vi "INI.GetSettings.vi"(8 "error in (no error)":errorcluster, 10 "INI Folder Location":path, 11 "State Variables":T1={"Events.State"=refnum, "Events.Test Result"=refnum, "Events.Progress"=refnum, "INI.Settings"={"Build Location"=path "C:/Simple Sequence Editor/SequenceRepo", "LoggingLocation"=path "", "Sequence.AbortChannel"="", "Sequence.IterationInfoChannel"="", "Sequence.DurationChannel"="", "Sequence.StepInfoChannel"="", "Sequence.SkipChannel"="", "PlotChannels"=[], "Sequence.InitializeScript"=path "C:/Simple Sequence Editor/SequenceRepo", "Sequence.CleanupScript"=path "", "Log.DefaultRate"=0.0}, "NIVS.AlarmManager"=refnum, "NIVS.BaseLogPath"=path "", "NIVS.DataLogManagerRef"=refnum, "NIVS.DataLogSpecRef"=refnum, "NIVS.Deployed"=FALSE, "NIVS.Events"={"SequenceEvent"=refnum, "SystemChangeEvent"=refnum, "WorkspaceEvent"=refnum}, "NIVS.GatewayIPAddress"="", "NIVS.DataLogGUID"="", "NIVS.ProfileCallback"=refnum, "NIVS.ProfileRef"=refnum, "NIVS.SequenceState"=enum."Idle", "NIVS.SystemDefinitionFile"=path "", "NIVS.SystemStateRefs"={"CustDatRef"=refnum, "EvtRef"=refnum, "Target State User Event"=refnum}, "NIVS.WorkspaceManager"=refnum, "NIVS.EventLogGUID"="", "NIVS.EventLogManagerRef"=refnum, "NIVS.EventLogSpecRef"=refnum, "NIVS.BaseToolPath"=path "", "Restart.Path"=path "", "Sequence.#ofColumns"=0, "Sequence.Iterations"=0, "Sequence.Channels"=[], "Sequence.ValidConfig?"=FALSE, "Station.ID"="", "UDP.Queue"=refnum, "UI.Abort"=refnum, "UI.Alarms"=refnum, "UI.Apply"=refnum, "UI.Back"=refnum, "UI.BaseFileName"=refnum, "UI.CurrentIteration"=refnum, "UI.CurrentStep"=refnum, "UI.CyclicFrequency"=refnum, "UI.Description"=refnum, "UI.DelayTime"=refnum, "UI.DisableAlarms"=refnum, "UI.Duration"=refnum, "UI.EnableLogging"=refnum, "UI.EnableState"=refnum, "UI.High"=refnum, "UI.LogChannels"=refnum, "UI.Low"=refnum, "UI.MonitoredVariable"=refnum, "UI.Next"=refnum, "UI.NumberOfCycles"=refnum, "UI.OperatorName"=refnum, "UI.Pause"=refnum, "UI.Profile"=refnum, "UI.Revert"=refnum, "UI.Skip"=refnum, "UI.Start"=refnum, "UI.StartIteration"=refnum, "UI.StartStep"=refnum, "UI.TabControl"=refnum, "UI.TotalIterations"=refnum, "UI.WaveformDefinition"=refnum, "UI.WaveformPreview"=refnum, "UI.WorkOrderNumber"=refnum, "UI.Chart"=refnum, "UI.Status"=refnum, "UI.DataView"=refnum, "UI.Table"=refnum, "UI.Multihead"=refnum, "UI.ToolTab"=refnum, "UI.Result"=refnum, "UI.Log Path"=refnum, "UI.ReportPath"=refnum, "UI.RestartPath"=refnum, "UI.AlarmLog"=refnum}) -> (0 "error out":errorcluster, 3 "INI.Settings":T2={"Build Location"=path "C:/Simple Sequence Editor/SequenceRepo", "LoggingLocation"=path "", "Sequence.AbortChannel"="", "Sequence.IterationInfoChannel"="", "Sequence.DurationChannel"="", "Sequence.StepInfoChannel"="", "Sequence.SkipChannel"="", "PlotChannels"=[], "Sequence.InitializeScript"=path "C:/Simple Sequence Editor/SequenceRepo", "Sequence.CleanupScript"=path "", "Log.DefaultRate"=0.0})   [LabVIEW 2015, in "Single Station Execution.lvlib"]
uses:
  Single Station Execution.lvlib
  Types/INI.Settings.ctl
  Types/Main.StateVariables.ctl
  <vilib>/NI Veristand/Execution/AlarmManager/AlarmManagerAPI.ctl
  NationalInstruments.VeriStand.ClientAPI
  <vilib>/NI Veristand/Execution/DataLogging/IDataLogging Ref.ctl
  <vilib>/NI Veristand/Execution/DataLogging/DataLoggingSpecification Ref.ctl
  Types/Execute.UserEventRefs.ctl
  <vilib>/NI Veristand/Execution/Workspace/SystemStateRegEventRef.ctl
  <vilib>/NI Veristand/Execution/Workspace/Target State Info.ctl
  <vilib>/NI Veristand/Execution/Workspace/Target State.ctl
  Types/Execution.SequenceState.ctl
  <vilib>/NI Veristand/Execution/Workspace/SystemStateEventRef.ctl
  <vilib>/NI Veristand/Execution/Workspace/WorkspaceAPI.ctl
  Types/UDPEngine.QueueCluster.ctl
  Types/UDPEngine.State.ctl
  Main.Constants.vi
  <vilib>/Utility/config.llb/Read Key (Path).vi
  <vilib>/Utility/config.llb/Write Key (Path).vi
  <vilib>/Utility/config.llb/Read Key (Double).vi
  <vilib>/Utility/config.llb/Write Key (Double).vi
  <vilib>/Utility/config.llb/Read Key (String).vi
  <vilib>/Utility/config.llb/Write Key (String).vi
  <vilib>/Utility/config.llb/NI_LVConfig.lvlib
  <vilib>/NI Veristand/Execution/Workspace/NI_VS Workspace ExecutionAPI.lvlib
  <vilib>/NI Veristand/Execution/DataLogging/NI_VS Data Logging API.lvlib
  <vilib>/NI Veristand/Execution/AlarmManager/NI_VS AlarmManager ExecutionAPI.lvlib
  NationalInstruments.VeriStand.RealTimeSequenceDefinitionApi
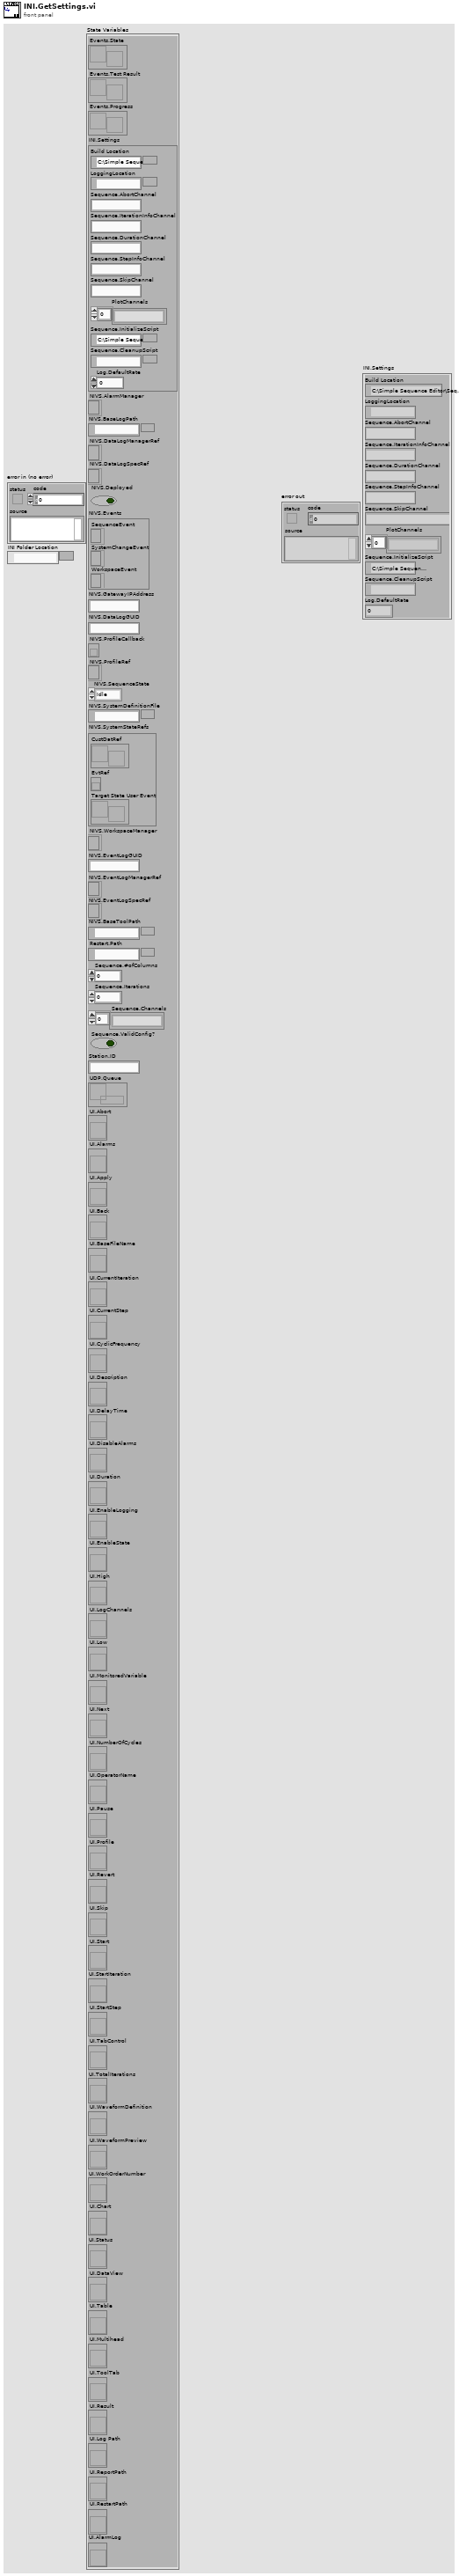
[diagram p1: front panel]
types:
  T1 = typedef "Single Station Execution.lvlib/Main.StateVariables.ctl" = cluster{"Events.State":refnum<user-event>, "Events.Test Result":refnum<user-event>, "Events.Progress":refnum<user-event>, "INI.Settings":T2, "NIVS.AlarmManager":T3, "NIVS.BaseLogPath":path, "NIVS.DataLogManagerRef":T4, "NIVS.DataLogSpecRef":T5, "NIVS.Deployed":bool, "NIVS.Events":T6, "NIVS.GatewayIPAddress":string, "NIVS.DataLogGUID":string, "NIVS.ProfileCallback":refnum<k27>, "NIVS.ProfileRef":refnum<k24>, "NIVS.SequenceState":T8, "NIVS.SystemDefinitionFile":path, "NIVS.SystemStateRefs":T9, "NIVS.WorkspaceManager":T10, "NIVS.EventLogGUID":string, "NIVS.EventLogManagerRef":T4, "NIVS.EventLogSpecRef":T5, "NIVS.BaseToolPath":path, "Restart.Path":path, "Sequence.#ofColumns":i32, "Sequence.Iterations":u32, "Sequence.Channels":string[], "Sequence.ValidConfig?":bool, "Station.ID":string, "UDP.Queue":refnum<queue>, "UI.Abort":refnum<vi>, "UI.Alarms":refnum<vi>, "UI.Apply":refnum<vi>, "UI.Back":refnum<vi>, "UI.BaseFileName":refnum<vi>, "UI.CurrentIteration":refnum<vi>, "UI.CurrentStep":refnum<vi>, "UI.CyclicFrequency":refnum<vi>, "UI.Description":refnum<vi>, "UI.DelayTime":refnum<vi>, "UI.DisableAlarms":refnum<vi>, "UI.Duration":refnum<vi>, "UI.EnableLogging":refnum<vi>, "UI.EnableState":refnum<vi>, "UI.High":refnum<vi>, "UI.LogChannels":refnum<vi>, "UI.Low":refnum<vi>, "UI.MonitoredVariable":refnum<vi>, "UI.Next":refnum<vi>, "UI.NumberOfCycles":refnum<vi>, "UI.OperatorName":refnum<vi>, "UI.Pause":refnum<vi>, "UI.Profile":refnum<vi>, "UI.Revert":refnum<vi>, "UI.Skip":refnum<vi>, "UI.Start":refnum<vi>, "UI.StartIteration":refnum<vi>, "UI.StartStep":refnum<vi>, "UI.TabControl":refnum<vi>, "UI.TotalIterations":refnum<vi>, "UI.WaveformDefinition":refnum<vi>, "UI.WaveformPreview":refnum<vi>, "UI.WorkOrderNumber":refnum<vi>, "UI.Chart":refnum<vi>, "UI.Status":refnum<vi>, "UI.DataView":refnum<vi>, "UI.Table":refnum<vi>, "UI.Multihead":refnum<vi>, "UI.ToolTab":refnum<vi>, "UI.Result":refnum<vi>, "UI.Log Path":refnum<vi>, "UI.ReportPath":refnum<vi>, "UI.RestartPath":refnum<vi>, "UI.AlarmLog":refnum<vi>}
  T2 = typedef "Single Station Execution.lvlib/INI.Settings.ctl" = cluster{"Build Location":path, "LoggingLocation":path, "Sequence.AbortChannel":string, "Sequence.IterationInfoChannel":string, "Sequence.DurationChannel":string, "Sequence.StepInfoChannel":string, "Sequence.SkipChannel":string, "PlotChannels":string[], "Sequence.InitializeScript":path, "Sequence.CleanupScript":path, "Log.DefaultRate":dbl}
  T3 = typedef "NI_VS AlarmManager ExecutionAPI.lvlib/AlarmManagerAPI.ctl" = refnum<k24>
  T4 = typedef "NI_VS Data Logging API.lvlib/IDataLogging Ref.ctl" = refnum<k24>
  T5 = typedef "NI_VS Data Logging API.lvlib/DataLoggingSpecification Ref.ctl" = refnum<k24>
  T6 = typedef "Single Station Execution.lvlib/Execute.UserEventRefs.ctl" = cluster{"SequenceEvent":refnum<event-registration>, "SystemChangeEvent":T7, "WorkspaceEvent":refnum<event-registration>}
  T7 = typedef "NI_VS Workspace ExecutionAPI.lvlib/SystemStateRegEventRef.ctl" = refnum<event-registration>
  T8 = typedef "Single Station Execution.lvlib/Execution.SequenceState.ctl" = enum16{"Idle", "Initializing", "Running", "Paused", "Finalizing", "Complete"}
  T9 = typedef "NI_VS Workspace ExecutionAPI.lvlib/SystemStateEventRef.ctl" = cluster{"CustDatRef":refnum<user-event>, "EvtRef":refnum<k27>, "Target State User Event":refnum<user-event>}
  T10 = typedef "NI_VS Workspace ExecutionAPI.lvlib/WorkspaceAPI.ctl" = refnum<k24>
  T11 = typedef "NI_LVConfig.lvlib/Config Data RefNum.ctl" = refnum<k1>
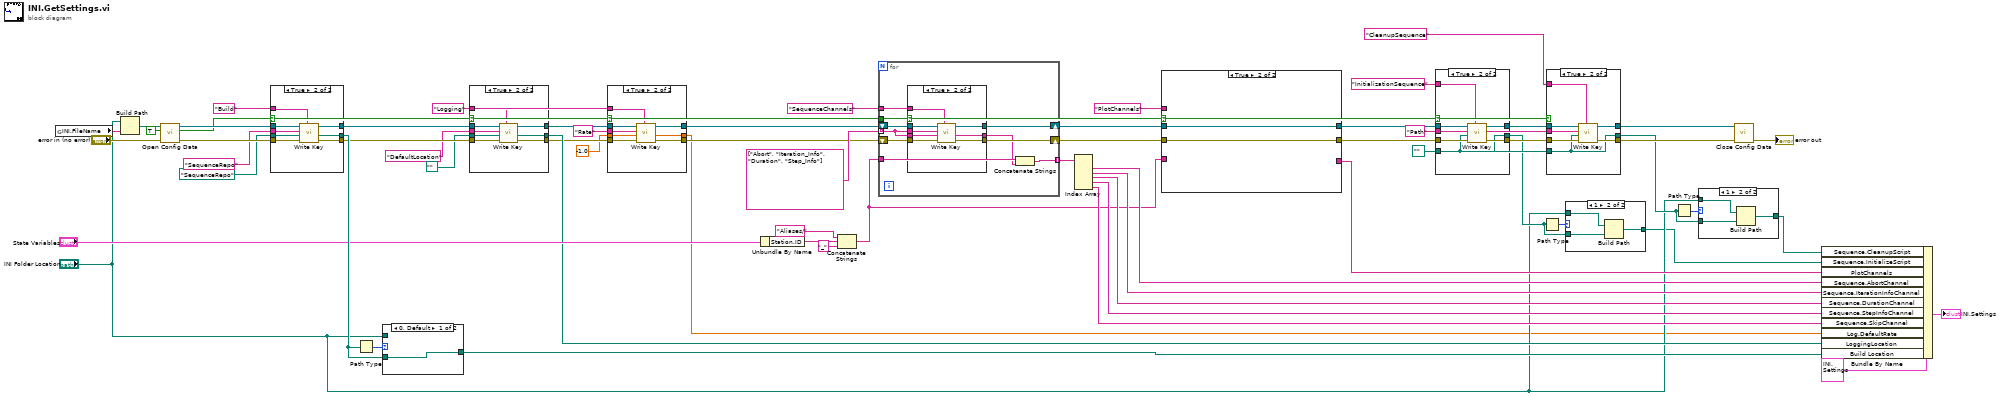
[diagram p0: block diagram]
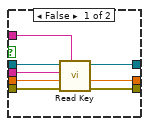
[diagram p2: hidden frame]
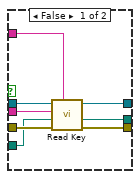
[diagram p5: hidden frame]
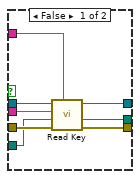
[diagram p6: hidden frame]
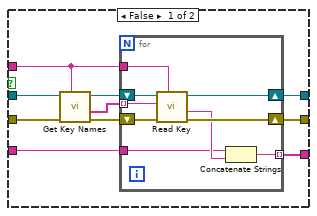
[diagram p7: hidden frame]
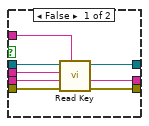
[diagram p8: hidden frame]
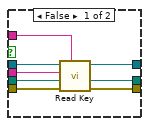
[diagram p9: hidden frame]
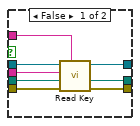
[diagram p10: hidden frame]
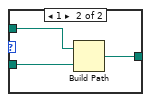
[diagram p11: hidden frame]
diagram:
  w22 = path "" ("default value")
  w18 = "Path" ("section")
  w6 = "Logging" ("section")
  n1 = global read "Main.Constants.vi" "INI.FileName"() -> (w55:string)
  n2 = Build Path(base path="INI Folder Location", name or relative path=w55) -> (appended path=w56:path)
  n3 = call <vilib>:"Open Config Data.vi"("error in (no error)"="error in (no error)", "create file if necessary (T)"=TRUE, "configuration file path"=w56) -> ("error out"=w62:errorcluster, "file created?"=w7:bool, "refnum"=w63:T11)  [unwired: 6 in]
  n4 = case shown="True" w7 {
    tunnel: w63 -> [w71 w76]
    tunnel: w62 -> [w70 w78]
    tunnel: [w69 w74] -> w48
    tunnel: [w68 w72] -> w46
    tunnel: "Build" ("section") -> [w67 w75]
    tunnel: "SequenceRepo" ("key") -> [w66 w77]
    tunnel: path "SequenceRepo" ("default value") -> [w65 w73]
    tunnel: [w64 w73] -> w57
    frame False {
      n5 = call-poly <vilib>:"Read Key.vi"("section"=w67, "error in (no error)"=w70, "default value"=w65, "key"=w66, "refnum"=w71) -> ("error out"=w69:errorcluster, "value"=w64:path, "refnum out"=w68:T11)  [unwired: 3 in, 1 out]
    }
    frame True {
      n6 = call-poly <vilib>:"Write Key.vi"("section"=w75, "error in (no error)"=w78, "value"=w73, "key"=w77, "refnum"=w76) -> ("error out"=w74:errorcluster, "refnum out"=w72:T11)  [unwired: 4 in, 1 out]
    }
  }
  n7 = Path Type(1:w57) -> (0:w58:i16)
  n8 = case shown="0, Default" w58 {
    tunnel: w57 -> [w79 w82]
    tunnel: [w79 w81] -> w50
    tunnel: "INI Folder Location" -> [_ w80]
    frame 0, Default {
    }
    frame 1 {
      n9 = Build Path(base path=w80, name or relative path=w82) -> (appended path=w81:path)
    }
  }
  n10 = case shown="True" w7 {
    tunnel: w46 -> [w90 w95]
    tunnel: w48 -> [w89 w97]
    tunnel: [w88 w93] -> w9
    tunnel: [w87 w91] -> w3
    tunnel: w6 -> [w86 w94]
    tunnel: "DefaultLocation" ("key") -> [w85 w96]
    tunnel: path "" ("default value") -> [w84 w92]
    tunnel: [w83 w92] -> w32
    frame False {
      n11 = call-poly <vilib>:"Read Key.vi"("section"=w86, "error in (no error)"=w89, "default value"=w84, "key"=w85, "refnum"=w90) -> ("error out"=w88:errorcluster, "value"=w83:path, "refnum out"=w87:T11)  [unwired: 3 in, 1 out]
    }
    frame True {
      n12 = call-poly <vilib>:"Write Key.vi"("section"=w94, "error in (no error)"=w97, "value"=w92, "key"=w96, "refnum"=w95) -> ("error out"=w93:errorcluster, "refnum out"=w91:T11)  [unwired: 4 in, 1 out]
    }
  }
  n13 = case shown="True" w7 {
    tunnel: w3 -> [w105 w110]
    tunnel: w9 -> [w104 w112]
    tunnel: [w103 w108] -> w8
    tunnel: [w102 w106] -> w2
    tunnel: w6 -> [w101 w109]
    tunnel: "Rate" ("key") -> [w100 w111]
    tunnel: -1.0 -> [w99 w107]
    tunnel: [w98 w107] -> w1
    frame False {
      n14 = call-poly <vilib>:"Read Key.vi"("section"=w101, "error in (no error)"=w104, "default value"=w99, "key"=w100, "refnum"=w105) -> ("error out"=w103:errorcluster, "value"=w98:dbl, "refnum out"=w102:T11)  [unwired: 3 in, 1 out]
    }
    frame True {
      n15 = call-poly <vilib>:"Write Key.vi"("section"=w109, "error in (no error)"=w112, "value"=w107, "key"=w111, "refnum"=w110) -> ("error out"=w108:errorcluster, "refnum out"=w106:T11)  [unwired: 4 in, 1 out]
    }
  }
  n16 = Unbundle By Name("State Variables") -> ("Station.ID"=w33:string)
  n17 = Concatenate Strings("Aliases/" ("string"), w33, "_" ("string")) -> (w29:string)
  n18 = for {
    tunnel: w7 -> [w122]
    tunnel: "SequenceChannels" ("section") -> [w117]
    shift-right: [w120] -> w31
    shift-left: w8 -> [w121]
    shift-right: [w119] -> w28
    shift-left: w2 -> [w118]
    tunnel: string[] ["Abort", "Iteration_Info", "Duration", "Step_Info"] -> [w115] mode=indexing
    tunnel: [w113] -> w42 mode=indexing
    tunnel: w29 -> [w116]
    n19 = case shown="True" w122 {
      tunnel: w118 -> [w130 w135]
      tunnel: w121 -> [w129 w137]
      tunnel: [w128 w133] -> w120
      tunnel: [w127 w131] -> w119
      tunnel: w117 -> [w126 w134]
      tunnel: w115 -> [w125 w136]
      tunnel: w115 -> [w124 w132]
      tunnel: [w123 w132] -> w114
      frame False {
        n20 = call-poly <vilib>:"Read Key.vi"("section"=w126, "error in (no error)"=w129, "default value"=w124, "key"=w125, "refnum"=w130) -> ("error out"=w128:errorcluster, "value"=w123:string, "refnum out"=w127:T11)  [unwired: 3 in, 1 out]
      }
      frame True {
        n21 = call-poly <vilib>:"Write Key.vi"("section"=w134, "error in (no error)"=w137, "value"=w132, "key"=w136, "refnum"=w135) -> ("error out"=w133:errorcluster, "refnum out"=w131:T11)  [unwired: 4 in, 1 out]
      }
    }
    n22 = Concatenate Strings(w116, w114) -> (w113:string)
  }
  n23 = Index Array(array=w42) -> (element #1=w41:string, element #2=w37:string, element #3=w38:string, element #4=w39:string, element #5=w40:string)  [unwired: 5 in]
  n24 = case shown="True" w7 {
    tunnel: w28 -> [w146 w157]
    tunnel: w31 -> [w145 w156]
    tunnel: [w142 w156] -> w26
    tunnel: [w139 w157] -> w25
    tunnel: "PlotChannels" ("section") -> [w144 _]
    tunnel: w29 -> [w140 _]
    tunnel: [w138 _] -> w27
    frame False {
      n25 = call <vilib>:"Get Key Names.vi"("section"=w144, "error in (no error)"=w145, "refnum"=w146) -> ("error out"=w142:errorcluster, "key names"=w143:string[], "refnum out"=w141:T11)  [unwired: 5 in, 1 out]
      n26 = for {
        tunnel: w144 -> [w155]
        tunnel: w143 -> [w154] mode=indexing
        shift-right: [w151] -> w139
        shift-left: w141 -> [w152]
        shift-right: [w150] -> _
        shift-left: w142 -> [w153]
        tunnel: w140 -> [w148]
        tunnel: [w147] -> w138 mode=indexing
        n27 = call-poly <vilib>:"Read Key.vi"("section"=w155, "error in (no error)"=w153, "key"=w154, "refnum"=w152) -> ("error out"=w150:errorcluster, "value"=w149:string, "refnum out"=w151:T11)  [unwired: 4 in, 1 out]
        n28 = Concatenate Strings(w148, w149) -> (w147:string)
      }
    }
    frame True {
    }
  }
  n29 = case shown="True" w7 {
    tunnel: w26 -> [w165 w172]
    tunnel: [w164 w171] -> w23
    tunnel: w25 -> [w163 w169]
    tunnel: [w162 w170] -> w19
    tunnel: "InitializationSequence" ("section") -> [w161 w168]
    tunnel: w18 -> [w160 w167]
    tunnel: w22 -> [w159 w166]
    tunnel: [w158 w166] -> w12
    frame False {
      n30 = call-poly <vilib>:"Read Key.vi"("section"=w161, "error in (no error)"=w165, "default value"=w159, "key"=w160, "refnum"=w163) -> ("error out"=w164:errorcluster, "value"=w158:path, "refnum out"=w162:T11)  [unwired: 3 in, 1 out]
    }
    frame True {
      n31 = call-poly <vilib>:"Write Key.vi"("section"=w168, "error in (no error)"=w172, "value"=w166, "key"=w167, "refnum"=w169) -> ("error out"=w171:errorcluster, "refnum out"=w170:T11)  [unwired: 4 in, 1 out]
    }
  }
  n32 = Path Type(1:w12) -> (0:w13:i16)
  n33 = case shown="True" w7 {
    tunnel: w23 -> [w180 w187]
    tunnel: [w179 w186] -> w21
    tunnel: w19 -> [w178 w184]
    tunnel: [w177 w185] -> w20
    tunnel: "CleanupSequence" ("section") -> [w176 w183]
    tunnel: w18 -> [w175 w182]
    tunnel: w22 -> [w174 w181]
    tunnel: [w173 w181] -> w15
    frame False {
      n34 = call-poly <vilib>:"Read Key.vi"("section"=w176, "error in (no error)"=w180, "default value"=w174, "key"=w175, "refnum"=w178) -> ("error out"=w179:errorcluster, "value"=w173:path, "refnum out"=w177:T11)  [unwired: 3 in, 1 out]
    }
    frame True {
      n35 = call-poly <vilib>:"Write Key.vi"("section"=w183, "error in (no error)"=w187, "value"=w181, "key"=w182, "refnum"=w184) -> ("error out"=w186:errorcluster, "refnum out"=w185:T11)  [unwired: 4 in, 1 out]
    }
  }
  n36 = case shown="1" w13 {
    tunnel: w12 -> [w188 w191]
    tunnel: [w188 w190] -> w10
    tunnel: "INI Folder Location" -> [_ w189]
    frame 0, Default {
    }
    frame 1 {
      n37 = Build Path(base path=w189, name or relative path=w191) -> (appended path=w190:path)
    }
  }
  n38 = Path Type(1:w15) -> (0:w16:i16)
  n39 = case shown="1" w16 {
    tunnel: w15 -> [w192 w195]
    tunnel: [w192 w194] -> w14
    tunnel: "INI Folder Location" -> [_ w193]
    frame 0, Default {
    }
    frame 1 {
      n40 = Build Path(base path=w193, name or relative path=w195) -> (appended path=w194:path)
    }
  }
  n41 = call <vilib>:"Close Config Data.vi"("error in (no error)"=w21, "refnum"=w20) -> ("error out"=→"error out":errorcluster)  [unwired: 8 in, 1 out]
  n42 = Bundle By Name(cluster=T2 {"Build Location"=path "C:/Simple Sequence Editor/SequenceRepo", "LoggingLocation"=path "", "Sequence.AbortChannel"="", "Sequence.IterationInfoChannel"="", "Sequence.DurationChannel"="", "Sequence.StepInfoChannel"="", "Sequence.SkipChannel"="", "PlotChannels"=[], "Sequence.InitializeScript"=path "C:/Simple Sequence Editor/SequenceRepo", "Sequence.CleanupScript"=path "", "Log.DefaultRate"=0.0}, "Sequence.CleanupScript"=w14, "Sequence.InitializeScript"=w10, "PlotChannels"=w27, "Sequence.AbortChannel"=w41, "Sequence.IterationInfoChannel"=w37, "Sequence.DurationChannel"=w38, "Sequence.StepInfoChannel"=w39, "Sequence.SkipChannel"=w40, "Log.DefaultRate"=w1, "LoggingLocation"=w32, "Build Location"=w50) -> (→"INI.Settings":T2)
